vi "_RT_Pub_AccessExpCondi.vi"(7 "Function":enum16{"Write", "Read"}(ring)=enum."Read", 8 "error in (no error)":errorcluster, 9 "NewExpVar in":variant, 10 "ClassName":string="Laser") -> (0 "error out":errorcluster, 1 "Time Stamp":timestamp, 3 "ExpCondi":T1=[{"Label"="Laser", "Value"=variant}, {"Label"="Pressure", "Value"=variant}, {"Label"="TMP", "Value"=variant}, {"Label"="Script", "Value"=variant}, {"Label"="Signal Remarks", "Value"=variant}, {"Label"="ExtAO", "Value"=variant}, {"Label"="ExtDO", "Value"=variant}, {"Label"="ExtDI", "Value"=variant}, {"Label"="D999", "Value"=variant}])   [LabVIEW 2016]
uses:
  PublicSubVI/Ctl/_ctl_RT_ExpCondi.ctl
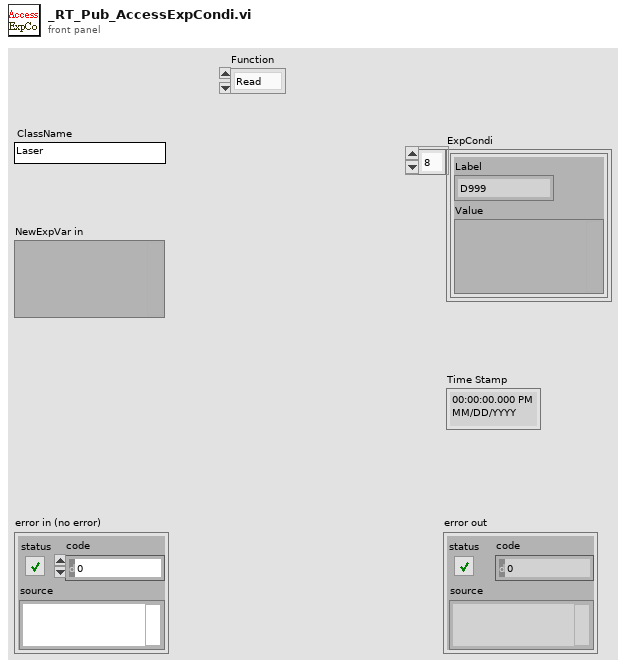
[diagram p1: front panel]
types:
  T1 = typedef "_ctl_RT_ExpCondi.ctl" = cluster{"Label":string, "Value":variant}[]
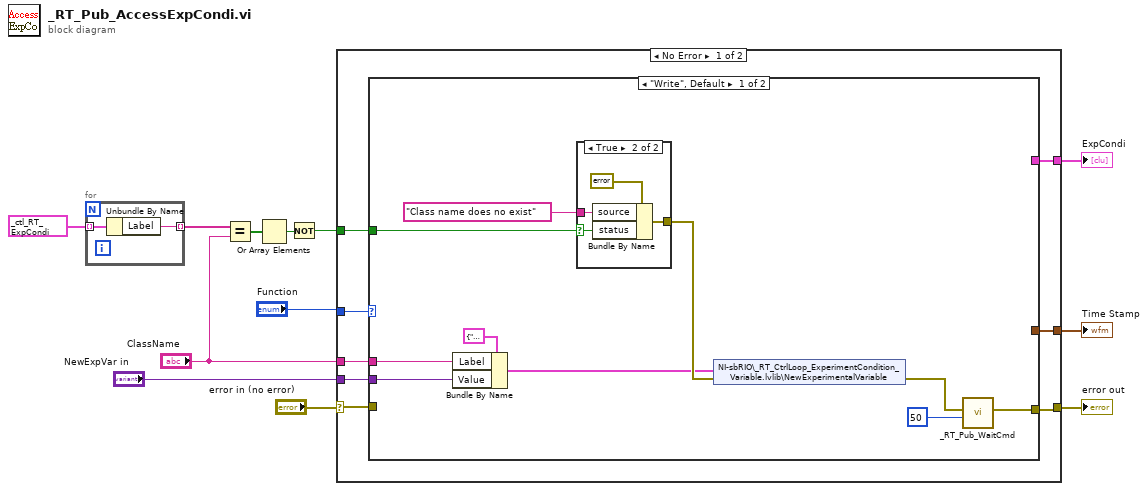
[diagram p0: block diagram]
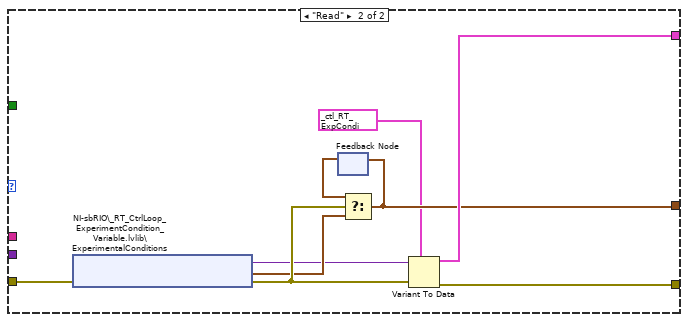
[diagram p3: hidden frame]
diagram:
  n1 = for {
    tunnel: T1 [{"Label"="Laser", "Value"=variant}, {"Label"="Pressure", "Value"=variant}, {"Label"="TMP", "Value"=variant}, {"Label"="Script", "Value"=variant}, {"Label"="Signal Remarks", "Value"=variant}, {"Label"="ExtAO", "Value"=variant}, {"Label"="ExtDO", "Value"=variant}, {"Label"="ExtDI", "Value"=variant}, {"Label"="DAQ", "Value"=variant}] ("ExpCondi") -> [w14] mode=indexing
    tunnel: [w13] -> w1 mode=indexing
    n2 = Unbundle By Name(w14) -> ("Label"=w13:string)
  }
  n3 = Equal?(x=w1, y="ClassName") -> (x = y?=w9:bool[])
  n4 = Or Array Elements(Boolean array=w9) -> (logical OR=w8:bool)
  n5 = Not(x=w8) -> (.not. x?=w4:bool)
  n6 = case shown="No Error" "error in (no error)" {
    selector: "error in (no error)" -> [w20 w46]
    tunnel: "Function" -> [w22 _]
    tunnel: [w21 _] -> w3
    tunnel: [w19 w46] -> w11
    tunnel: [w18 _] -> w10
    tunnel: "ClassName" -> [w17 _]
    tunnel: "NewExpVar in" -> [w16 _]
    tunnel: w4 -> [w15 _]
    frame No Error {
      n7 = case shown="\"Write\", Default" w22 {
        tunnel: [_ w45] -> w21
        tunnel: w20 -> [_ w44]
        tunnel: [w24 w43] -> w19
        tunnel: [_ w38] -> w18
        tunnel: w17 -> [w31 _]
        tunnel: w16 -> [w30 _]
        tunnel: w15 -> [w29 _]
        frame "Write", Default {
          n8 = Bundle By Name(cluster=cluster{"Label":string, "Value":variant} {"Label"="Laser", "Value"=variant} ("element"), "Label"=w31, "Value"=w30) -> (w26:cluster{"Label":string, "Value":variant})
          n9 = case shown="True" w29 {
            selector: w29 -> [_ w34]
            tunnel: [_ w35] -> w27
            tunnel: "Class name does no exist" -> [_ w33]
            frame False {
            }
            frame True {
              n10 = Bundle By Name(cluster=errorcluster {"status"=FALSE, "code"=0, "source"=""} ("error in"), "source"=w33, "status"=w34) -> (w35:errorcluster)
            }
          }
          n11 = shared-variable "NI-sbRIO\\_RT_CtrlLoop_ExperimentCondition_Variable.lvlib\\NewExperimentalVariable"(w26, error in=w27) -> (error out=w25:errorcluster)
          n12 = call "_RT_Pub_WaitCmd.vi"("milliseconds to wait"=u32 50, "error in (no error)"=w25) -> ("error out"=w24:errorcluster)  [unwired: 9 in]
        }
        frame "Read" {
          n13 = shared-variable "NI-sbRIO\\_RT_CtrlLoop_ExperimentCondition_Variable.lvlib\\ExperimentalConditions"(error in=w44) -> (w39:variant, error out=w42:errorcluster, w41:timestamp)
          n14 = feedback #1() -> (w40:timestamp)  [unwired: 1 in]
          n15 = Select(t=w40, s=w42, f=w41) -> (s? t:f=w38:timestamp)
          n16 = feedback-in #1(w38) -> ()
          n17 = Variant To Data(error in=w42, type=T1 [{"Label"="Laser", "Value"=variant}, {"Label"="Pressure", "Value"=variant}, {"Label"="TMP", "Value"=variant}, {"Label"="Script", "Value"=variant}, {"Label"="Signal Remarks", "Value"=variant}, {"Label"="ExtAO", "Value"=variant}, {"Label"="ExtDO", "Value"=variant}, {"Label"="ExtDI", "Value"=variant}, {"Label"="DAQ", "Value"=variant}] ("ExpCondi"), Variant=w39) -> (data=w45:T1, error out=w43:errorcluster)
        }
      }
    }
    frame Error {
    }
  }
  "error out" <- w11
  "Time Stamp" <- w10
  "ExpCondi" <- w3
